vi "Script Count Helper Loops.vi"(8 "error in":errorcluster, 10 "appended path":path, 11 "Application in":refnum<vi>) -> (0 "error out":errorcluster, 2 "Number of HL":string, 3 "VI out":refnum<vi>)   [LabVIEW 2019, in "Panther Dashboard.lvlib"]
uses:
  Panther Dashboard.lvlib
  <vilib>/Utility/traverseref.llb/TRef TravTarget.ctl
  <vilib>/Utility/traverseref.llb/VI Scripting - Traverse.lvlib
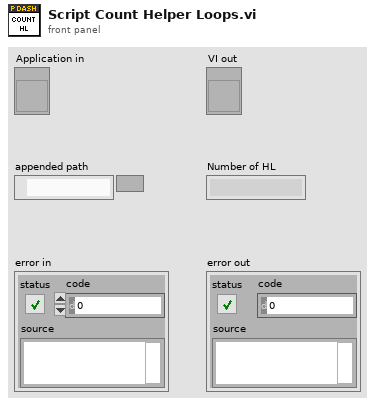
[diagram p1: front panel]
types:
  T1 = typedef "TRef TravTarget.ctl" = enum16{"FP", "BD", "Other"}
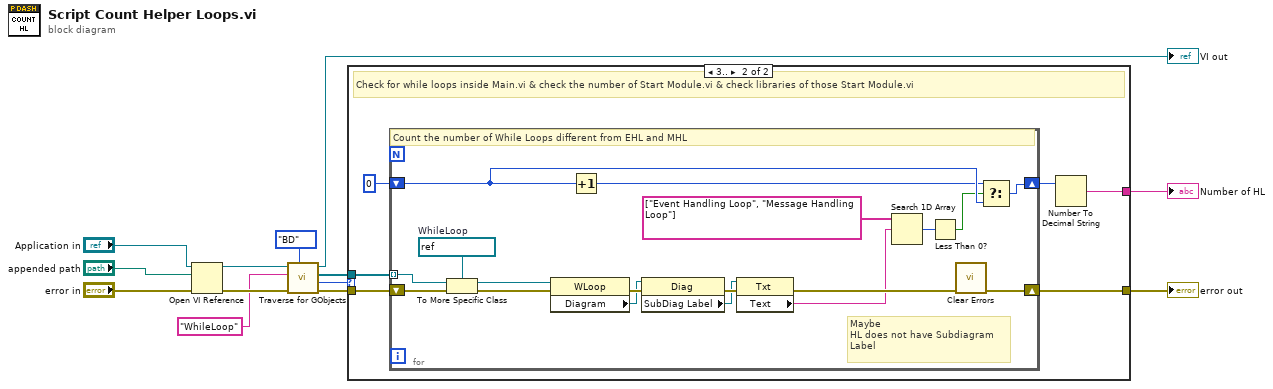
[diagram p0: block diagram]
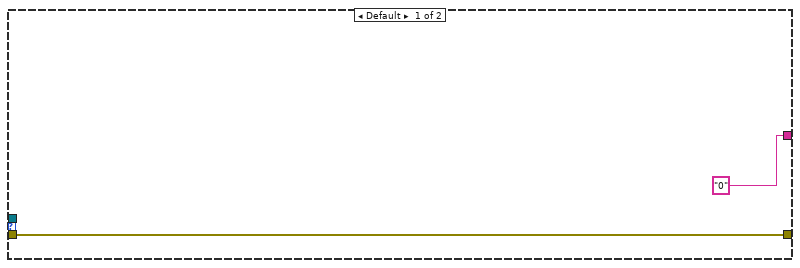
[diagram p2: hidden frame]
diagram:
  n1 = Open VI Reference(application reference (local)="Application in", vi path="appended path", error in (no error)="error in") -> (vi reference=w5:refnum<vi>, error out=w12:errorcluster)  [unwired: 3 in]
  n2 = call <vilib>:"Traverse for GObjects.vi"("Traverse Target"=TRef_TravTarget."BD", "error in (no error)"=w12, "Class Name"="WhileLoop", "VI Refnum"=w5) -> ("error out"=w10:errorcluster, "# of Refs"=w8:i32, "References"=w3:refnum<vi>[], "dup VI Refnum"=→"VI out":refnum<vi>)  [unwired: 4 in]
  n3 = case shown="3.." w8 {
    tunnel: w10 -> [w15 w21]
    tunnel: w3 -> [_ w19]
    tunnel: [w15 w20] -> w13
    tunnel: ["0" w16] -> w1
    frame Default {
    }
    frame 3.. {
      # "Check for while loops inside Main.vi & check the number of Start Module.vi & check libraries of those Start Module.vi"
      n4 = for {
        tunnel: w19 -> [w33] mode=indexing
        shift-right: [w34] -> w20
        shift-left: w21 -> [w39]
        shift-right: [w26] -> w17
        shift-left: 0 -> [w28]
        w32 = refnum<vi> refnum  # WhileLoop
        # "Maybe\nHL does not have Subdiagram\nLabel"
        # "Count the number of While Loops different from EHL and MHL"
        n5 = To More Specific Class(target class=w32, reference=w33, error in=w39) -> (specific class reference=w31:refnum<vi>, error out=w38:errorcluster)
        n6 = property class="WLoop"(reference=w31, error in=w38) -> (error out=w37:errorcluster, "Diagram"=w30:refnum<vi>)  [unwired: 1 out]
        n7 = Increment(x=w28) -> (x+1=w27:i32)
        n8 = property class="Diag"(reference=w30, error in=w37) -> (error out=w36:errorcluster, "SubDiag Label"=w29:refnum<vi>)  [unwired: 1 out]
        n9 = property class="Txt"(reference=w29, error in=w36) -> (error out=w35:errorcluster, "Text"=w24:string)  [unwired: 1 out]
        n10 = Search 1D Array(1D array=string[] ["Event Handling Loop", "Message Handling Loop"] ("y"), element=w24) -> (index of element=w23:i32)  [unwired: 1 in]
        n11 = Less Than 0?(x=w23) -> (x < 0?=w22:bool)
        n12 = call <vilib>:"Clear Errors.vi"("error in (no error)"=w35) -> ("error out"=w34:errorcluster)  [unwired: 5 in, 1 out]
        n13 = Select(t=w27, s=w22, f=w28) -> (s? t:f=w26:i32)
      }
      n14 = Number To Decimal String(number=w17) -> (decimal integer string=w16:string)  [unwired: 1 in]
    }
  }
  "error out" <- w13
  "Number of HL" <- w1
